vi "Get Human Readable Error.vi"(8 "error in (no error)":errorcluster) -> (2 "Error Message":string)   [LabVIEW 2021, in "CIF_UI.lvclass"]
uses:
  CIF_UI.lvclass
  <vilib>/CIF Foundation/CIF Utilities/Errors/Errors_CIF_U.lvlib
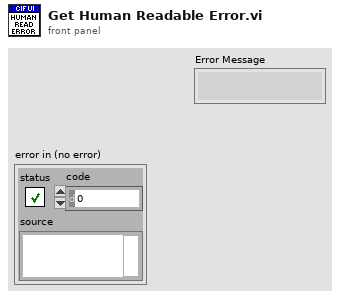
[diagram p1: front panel]
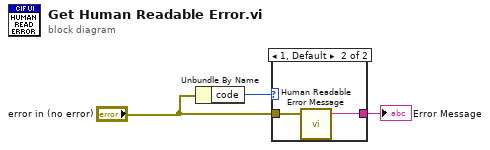
[diagram p0: block diagram]
diagram:
  n1 = Unbundle By Name("error in (no error)") -> ("code"=w3:i32)
  n2 = case shown="1, Default" w3 {
    tunnel: "error in (no error)" -> [_ w5]
    tunnel: [_ w4] -> w1
    frame 0 {
    }
    frame 1, Default {
      n3 = call <vilib>:"Human Readable Error Message.vi"("error in (no error)"=w5) -> ("Human readable error message"=w4:string)  [unwired: 4 in]
    }
  }
  "Error Message" <- w1
